vi "WAPIAerInitialize.vi"(0 "lpsParam":path, 2 "lpsFirm":path, 3 "lpsConfig":path, 9 "error in (no error)":errorcluster) -> (6 "error out":errorcluster)   [LabVIEW 2009]
uses:
  win50032.dll
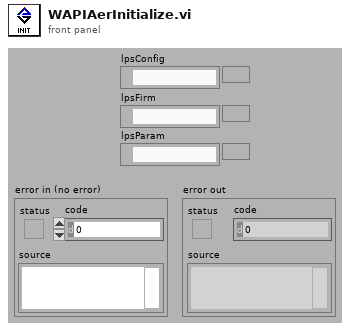
[diagram p1: front panel]
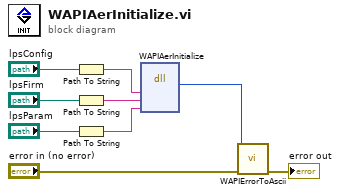
[diagram p0: block diagram]
diagram:
  n1 = Path To String(path="lpsConfig") -> (string=w3:string)
  n2 = Path To String(path="lpsFirm") -> (string=w2:string)
  n3 = Path To String(path="lpsParam") -> (string=w1:string)
  n4 = dll-call lib="win50032.dll" fn="WAPIAerInitialize"("lpsConfig"=w3, "lpsFirm"=w2, "lpsParam"=w1) -> ("return type"=w9:u32)  [unwired: 6 in, 2 out]
  n5 = call "WAPIErrorToAscii.vi"("error in (no error)"="error in (no error)", "error"=w9) -> ("error out"=→"error out":errorcluster)  [unwired: 8 in, 1 out]
